vi "test error before assertion.vi"(8 "error in (no error)":errorcluster, 11 "TestCase in":refnum<class "VI Test Comparison.lvclass">=refnum) -> (0 "error out":errorcluster, 3 "TestCase out":refnum<class "VI Test Comparison.lvclass">)   [LabVIEW 2020, in "VI Test Comparison.lvclass"]
uses:
  VI Test Comparison.lvclass
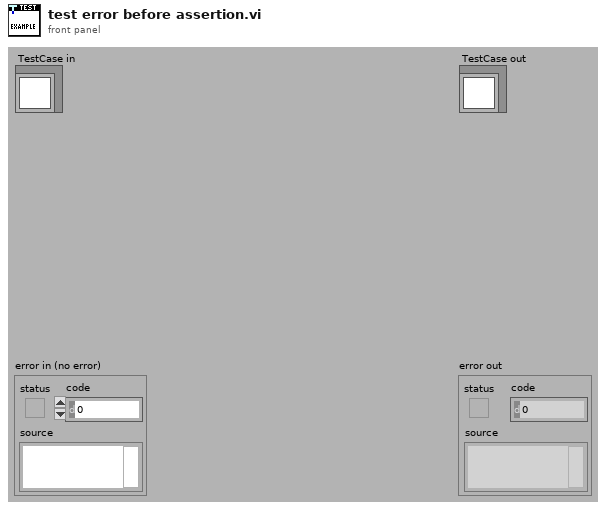
[diagram p1: front panel]
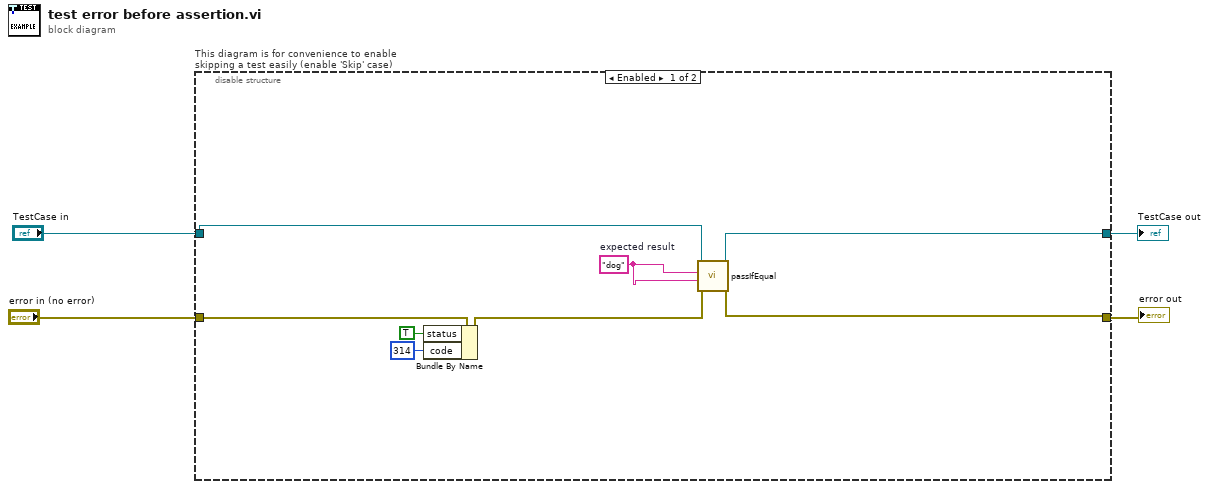
[diagram p0: block diagram]
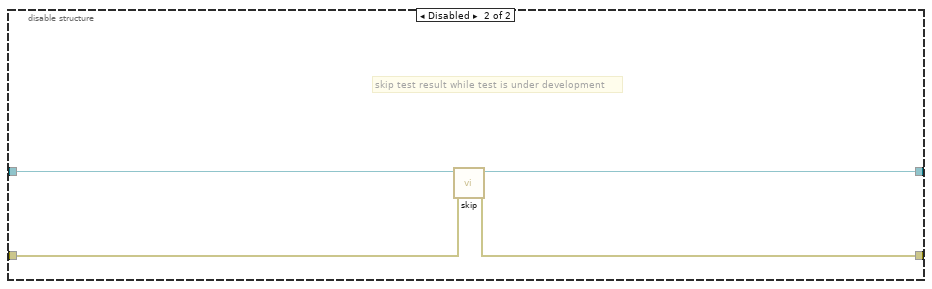
[diagram p2: hidden frame]
diagram:
  n1 = disable-structure "This diagram is for convenience to enable skipping a test easily (enable 'Skip' case)" shown="Enabled" {
    disable-tunnel: "TestCase in" -> [w12 w16]
    disable-tunnel: [w11 w14] -> w1
    disable-tunnel: [w10 w15] -> w3
    disable-tunnel: "error in (no error)" -> [w8 w13]
    frame Enabled {
      w9 = "dog"  # expected result
      n2 = Bundle By Name(cluster=w8, "status"=TRUE, "code"=314) -> (w7:errorcluster)
      n3 = call-dynamic "passIfEqual.vi"("error in (no error)"=w7, "y"=w9, "x"=w9, "TestCase in"=w12) -> ("error out"=w10:errorcluster, "TestCase out"=w11:refnum<class "VI Test Comparison.lvclass">)  [unwired: 6 in]
    }
    frame Disabled {
      # "skip test result while test is under development"
      n4 = call <vilib>:"skip.vi"("error in (no error)"=w13, "TestCase in"=w16) -> ("error out"=w15:errorcluster, "TestCase out"=w14:refnum<class "VI Test Comparison.lvclass">)  [unwired: 8 in]
    }
  }
  "error out" <- w3
  "TestCase out" <- w1
